vi "start.vi"(6 "timeout ms (5000)":i32=5000, 8 "error in (no error)":errorcluster, 11 "TCP Network Connection in":refnum<k5>) -> (0 "error out":errorcluster, 1 "Timeout?":bool, 3 "TCP Network Connection out":refnum<k5>)   [LabVIEW 2025, in "Newtons4thEkg.lvlib"]
uses:
  Newtons4thEkg.lvlib
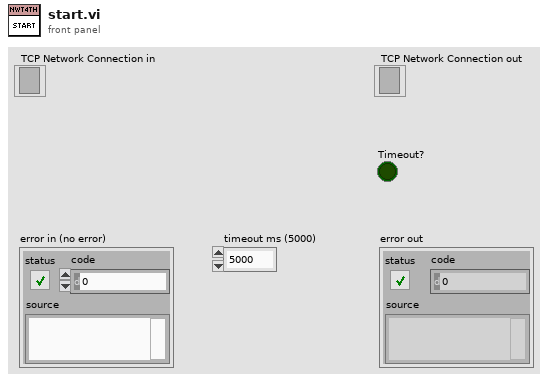
[diagram p1: front panel]
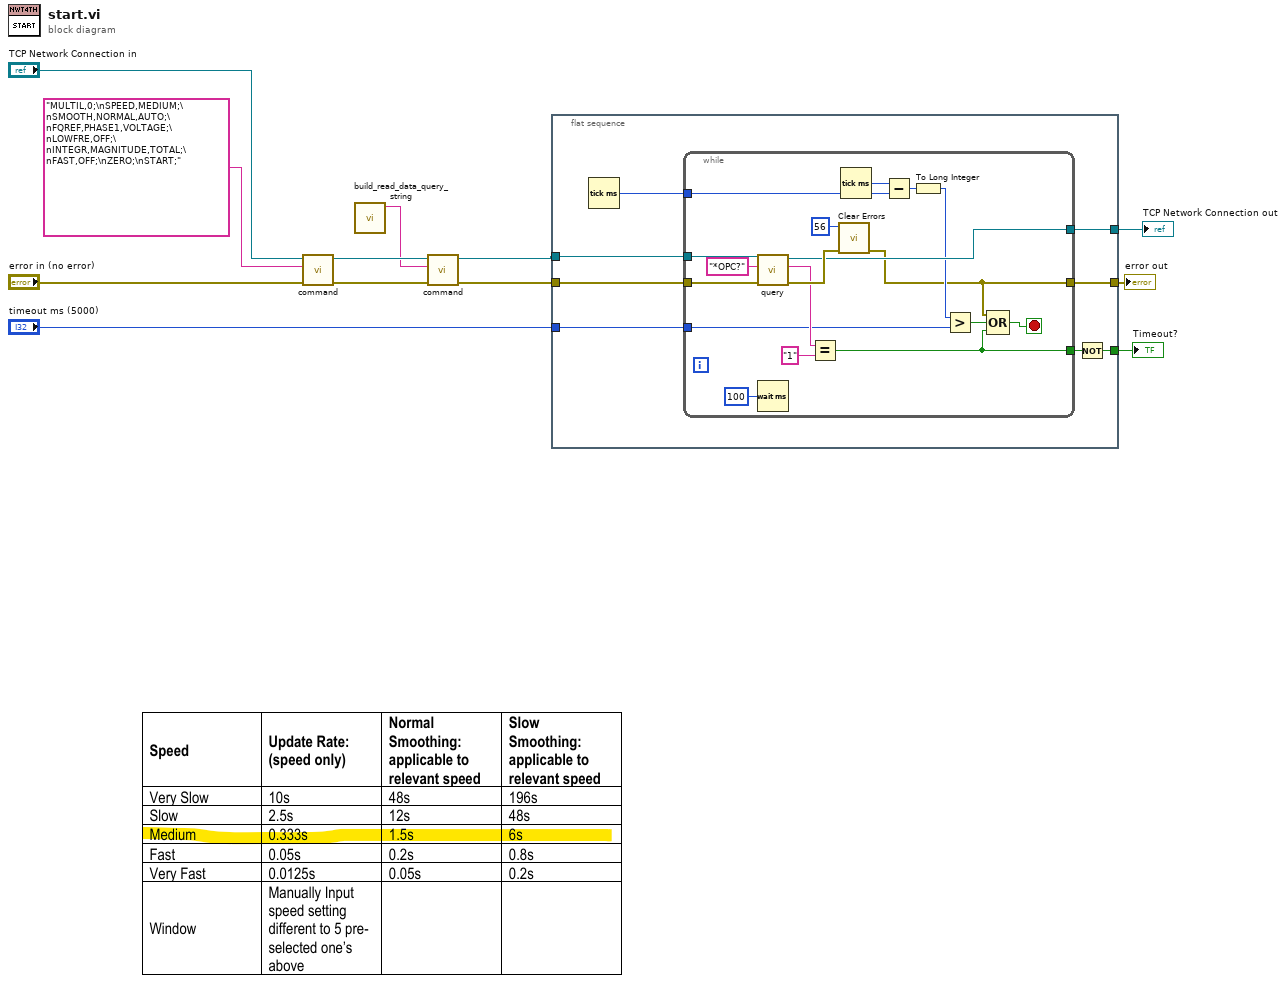
[diagram p0: block diagram]
diagram:
  n1 = call "command.vi"("error in (no error)"="error in (no error)", "Query"="MULTIL,0;\nSPEED,MEDIUM;\nSMOOTH,NORMAL,AUTO;\nFQREF,PHASE1,VOLTAGE;\nLOWFRE,OFF;\nINTEGR,MAGNITUDE,TOTAL;\nFAST,OFF;\nZERO;\nSTART;", "TCP in"="TCP Network Connection in") -> ("error out"=w11:errorcluster, "TCP out"=w8:refnum<k5>)  [unwired: 7 in]
  n2 = call "build_read_data_query_string.vi"() -> ("Query String"=w7:string)  [unwired: 11 in]
  n3 = call "command.vi"("error in (no error)"=w11, "Query"=w7, "TCP in"=w8) -> ("error out"=w6:errorcluster, "TCP out"=w3:refnum<k5>)  [unwired: 7 in]
  n4 = flat-sequence {
    tunnel: w6 -> [w20]
    tunnel: [w19] -> w5
    tunnel: [w18] -> w4
    tunnel: w3 -> [w17]
    tunnel: "timeout ms (5000)" -> [w16]
    tunnel: [w13] -> w1
    frame #0 {
      n5 = Tick Count (ms)() -> (millisecond timer value=w15:u32)
      n6 = while {
        tunnel: w20 -> [w38]
        tunnel: [w21] -> w19
        tunnel: [w35] -> w18
        tunnel: w17 -> [w36]
        tunnel: w16 -> [w26]
        tunnel: w15 -> [w27]
        tunnel: [w23] -> w14
        stop <- w30 stop-if-true
        n7 = call "query.vi"("error in (no error)"=w38, "Query"="*OPC?", "TCP in"=w36) -> ("error out"=w37:errorcluster, "Return String"=w32:string, "TCP out"=w35:refnum<k5>)  [unwired: 6 in]
        n8 = Wait (ms)(milliseconds to wait=u32 100) -> ()  [unwired: 1 out]
        n9 = Equal?(x=w32, y="1") -> (x = y?=w23:bool)
        n10 = call <vilib>:"Clear Errors.vi"("error in (no error)"=w37, "specific error code to clear (0: all)"=56) -> ("error out"=w21:errorcluster)  [unwired: 4 in, 1 out]
        n11 = Tick Count (ms)() -> (millisecond timer value=w28:u32)
        n12 = Subtract(x=w28, y=w27) -> (x-y=w25:u32)
        n13 = To Long Integer(number=w25) -> (32bit integer=w24:i32)
        n14 = Greater?(x=w24, y=w26) -> (0:w22:bool)
        n15 = Compound Arithmetic op=OR(w21, w22, w23) -> (w30:bool)
      }
      n16 = Not(x=w14) -> (.not. x?=w13:bool)
    }
  }
  "error out" <- w5
  "TCP Network Connection out" <- w4
  "Timeout?" <- w1
